vi "Generate_Coordinates.vi"(0 "location":T1(ring), 2 "saved x":i32, 3 "saved y":i32, 5 "error in (no error)":errorcluster) -> (16 "generated coordinates":cluster{"X":sgl, "Y":sgl}, 19 "error IO":errorcluster)   [LabVIEW 2020]
doc: "Generates random coordinates to simulate location of the book."
panel:
  # "select type of coordinate you want to generate:"
  # "for near saved location, enter saved x and y:"
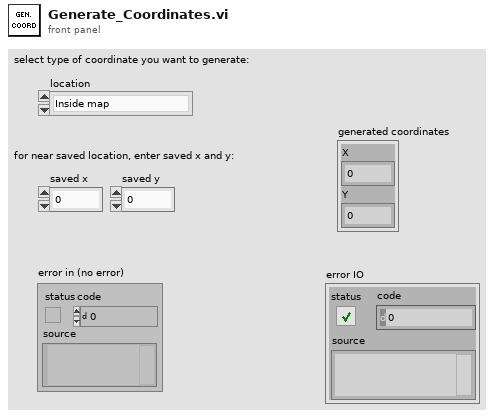
[diagram p1: front panel]
types:
  T1 = enum16{"Inside map", "Anywhere", "Near saved location"}
  T2 = typedef "Image_Cluster.ctl" = cluster{"Detector_info":cluster{"No. of detectors":dbl, "Detector_Array":string[][], "Detector_Array_Numeric":dbl[][]}, "Corner_info":cluster{"Corner_Array":dbl[][]}, "ROI":cluster{"Corners":cluster{"Global Rectangle":i32[], "Contours":cluster{"ID":enum32{"External", "Internal"}, "Type":u32, "Coordinates":i32[]}[]}[], "Detectors":cluster{"Global Rectangle":i32[], "Contours":cluster{"ID":enum32{"External", "Internal"}, "Type":u32, "Coordinates":i32[]}[]}[]}, "Shape_Detect":cluster{"Match_score":dbl, "Curve Parameters":T3, "Match Options":T4, "Circle Descriptor":cluster{"Min Radius":dbl, "Max Radius":dbl}}, "Path":cluster{"Config":path, "Map":path}, "Map":cluster{"X_resolution":i32, "Y_resolution":i32, "Image":T6}, "Conversion_factor":dbl}
  T3 = typedef "IMAQ Curve Parameters.ctl" = cluster{"Extraction Mode":u32, "Edge Threshold":i32, "Edge Filter Size":u32, "Min Length":i32, "Row Search Step Size":i32, "Col Search Step Size":i32, "Max Endpoint Gap":i32, "Closed":bool, "Subpixel":bool}
  T4 = typedef "ShapeDetectionMatchOptions.ctl" = cluster{"Rotation":bool, "Scale":bool, "Occlusion":bool, "Range Settings":T5[]}
  T5 = typedef "IMAQ Match Range Setting.ctl" = cluster{"Match Constraints":u32, "Min":dbl, "Max":dbl}
  T6 = typedef "IMAQ Image.ctl" = refnum<image>
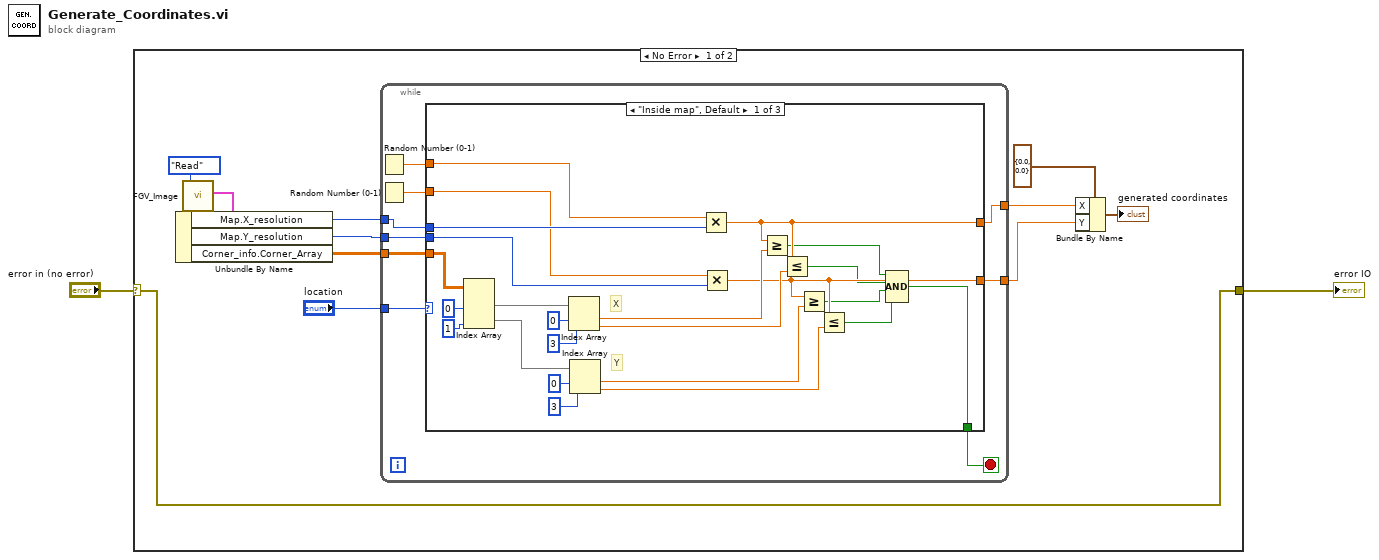
[diagram p0: block diagram]
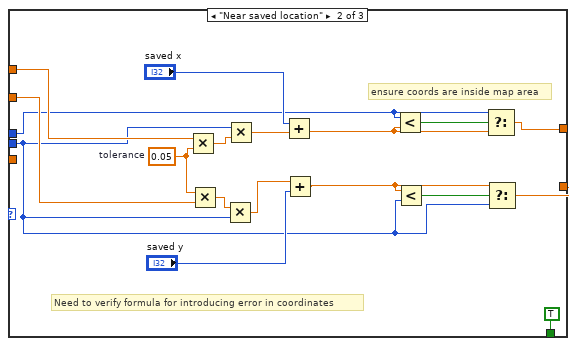
[diagram p2: hidden frame]
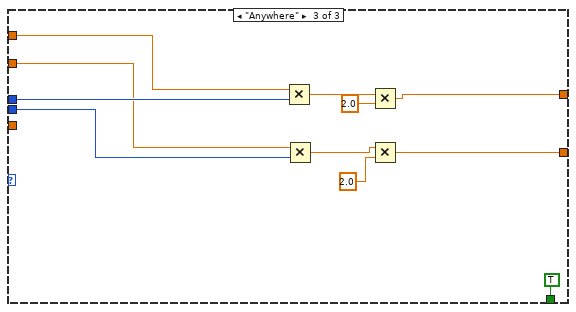
[diagram p3: hidden frame]
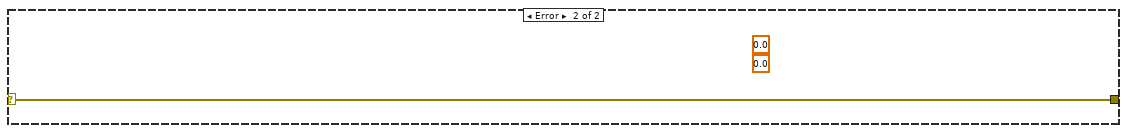
[diagram p4: hidden frame]
diagram:
  n1 = case shown="No Error" "error in (no error)" {
    selector: "error in (no error)" -> [w12 w76]
    tunnel: [w12 w76] -> w1
    frame No Error {
      n2 = call "FGV_Image.vi"("Action"=enum16{"Read", "Write", ""}."Read") -> ("Image_Cluster_out"=w10:T2)  [unwired: 10 in]
      n3 = Unbundle By Name(w10) -> ("Map.X_resolution"=w9:i32, "Map.Y_resolution"=w8:i32, "Corner_info.Corner_Array"=w3:dbl[][])
      n4 = while {
        tunnel: "location" -> [w22]
        tunnel: w9 -> [w19]
        tunnel: w8 -> [w18]
        tunnel: [w17] -> w6
        tunnel: [w16] -> w5
        tunnel: w3 -> [w15]
        stop <- w14 stop-if-true
        n5 = Random Number (0-1)() -> (number: 0 to 1=w21:dbl)
        n6 = Random Number (0-1)() -> (number: 0 to 1=w20:dbl)
        n7 = case shown="\"Inside map\", Default" w22 {
          tunnel: [w34 w52 w69] -> w17
          tunnel: [w31 w48 w67] -> w16
          tunnel: w19 -> [w46 w55 w75]
          tunnel: w18 -> [w45 w49 w74]
          tunnel: w21 -> [w44 w64 w73]
          tunnel: w20 -> [w43 w61 w72]
          tunnel: w15 -> [w39 _ _]
          tunnel: [w25 TRUE TRUE] -> w14
          frame "Inside map", Default {
            # "Y"
            # "X"
            n8 = Index Array(array=w39, index (col) #1=0 ("disabled index (col)"), index (col) #2=1 ("index (col)")) -> (element #1=w42:dbl[], element #2=w36:dbl[])  [unwired: 2 in]
            n9 = Index Array(array=w42, index #1=0 ("index"), index #2=3 ("index")) -> (element #1=w35:dbl, element #2=w33:dbl)
            n10 = Index Array(array=w36, index #1=0 ("index"), index #2=3 ("index")) -> (element #1=w32:dbl, element #2=w30:dbl)
            n11 = Multiply(x=w44, y=w46) -> (x*y=w34:dbl)
            n12 = Multiply(x=w43, y=w45) -> (x*y=w31:dbl)
            n13 = Greater Or Equal?(x=w34, y=w35) -> (x >= y?=w29:bool)
            n14 = Less Or Equal?(x=w34, y=w33) -> (x <= y?=w28:bool)
            n15 = Greater Or Equal?(x=w31, y=w32) -> (x >= y?=w27:bool)
            n16 = Less Or Equal?(x=w31, y=w30) -> (x <= y?=w26:bool)
            n17 = Compound Arithmetic op=AND(w29, w28, w27, w26) -> (w25:bool)
          }
          frame "Near saved location" {
            w62 = 0.05  # tolerance
            # "ensure coords are inside map area"
            # "Need to verify formula for introducing error in coordinates"
            n18 = Multiply(x=w64, y=w62) -> (x*y=w58:dbl)
            n19 = Multiply(x=w62, y=w61) -> (x*y=w59:dbl)
            n20 = Multiply(x=w59, y=w49) -> (x*y=w56:dbl)
            n21 = Multiply(x=w49, y=w58) -> (x*y=w57:dbl)
            n22 = Add(x="saved x", y=w57) -> (x+y=w53:dbl)
            n23 = Add(x=w56, y="saved y") -> (x+y=w50:dbl)
            n24 = Less?(x=w55, y=w53) -> (x < y?=w54:bool)
            n25 = Less?(x=w50, y=w49) -> (x < y?=w51:bool)
            n26 = Select(t=w55, s=w54, f=w53) -> (s? t:f=w52:dbl)
            n27 = Select(t=w50, s=w51, f=w49) -> (s? t:f=w48:dbl)
          }
          frame "Anywhere" {
            n28 = Multiply(x=w73, y=w75) -> (x*y=w71:dbl)
            n29 = Multiply(x=w72, y=w74) -> (x*y=w66:dbl)
            n30 = Multiply(x=w71, y=2.0) -> (x*y=w69:dbl)
            n31 = Multiply(x=w66, y=2.0) -> (x*y=w67:dbl)
          }
        }
      }
      n32 = Bundle By Name(cluster=cluster{"X":sgl, "Y":sgl} {"X"=0.0, "Y"=0.0}, "X"=w6, "Y"=w5) -> (→"generated coordinates":cluster{"X":sgl, "Y":sgl})
    }
    frame Error {
      (unwired) 0.0 ("Y Resolution")
      (unwired) 0.0 ("Y Resolution")
    }
  }
  "error IO" <- w1
